vi "Write Message Box.vi"(5 "Message Box":refnum<vi>, 9 "MessageBox in":refnum<class "MessageBox.lvclass">) -> (3 "MessageBox out":refnum<class "MessageBox.lvclass">)   [LabVIEW 2014, in "MessageBox.lvclass"]
uses:
  MessageBox.lvclass
  MessageBox.lvclass/MessageBox.ctl
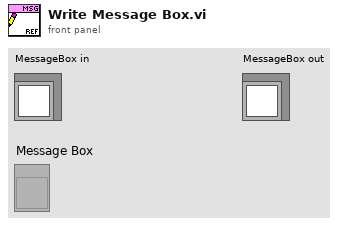
[diagram p1: front panel]
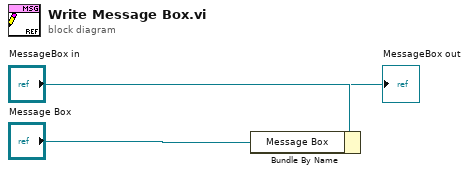
[diagram p0: block diagram]
diagram:
  n1 = Bundle By Name(cluster="MessageBox in", "Message Box"="Message Box") -> (→"MessageBox out":refnum<class "MessageBox.lvclass">)
